vi "PV Telegram return.vi"(4 "String received":string, 5 "Data Typ String":string) -> (0 "error":bool, 1 "Substring":string, 2 "PV Protocol Data out":string)   [LabVIEW 2018, in "Pfeiffer Vacuum.lvlib"]
uses:
  Pfeiffer Vacuum.lvlib
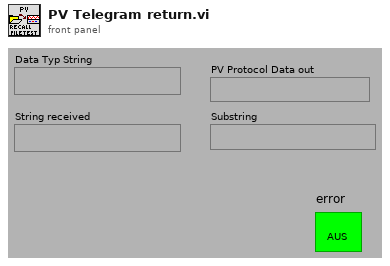
[diagram p1: front panel]
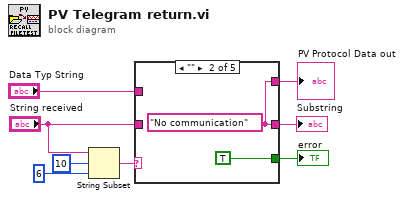
[diagram p0: block diagram]
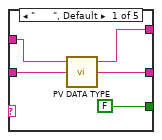
[diagram p2: hidden frame]
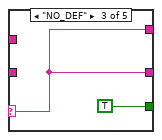
[diagram p3: hidden frame]
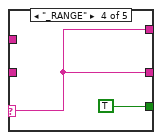
[diagram p4: hidden frame]
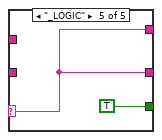
[diagram p5: hidden frame]
diagram:
  n1 = String Subset(string="String received", offset (0)=10 ("Offset (0)"), length (rest)=6 ("Länge")) -> (substring=w6:string)
  n2 = case shown="\"\"" w6 {
    selector: w6 -> [_ _ w16 w18 w20]
    tunnel: [w12 w14 w16 w18 w20] -> w7
    tunnel: "String received" -> [w13 _ _ _ _]
    tunnel: [FALSE TRUE TRUE TRUE TRUE] -> w3
    tunnel: "Data Typ String" -> [w10 _ _ _ _]
    tunnel: [w9 w14 w16 w18 w20] -> w1
    frame "      ", Default {
      n3 = call "PV DATA TYPE.vi"("String in"=w13, "Data Typ String in"=w10) -> ("Substring"=w12:string, "PV Protocol Data out"=w9:string)  [unwired: 2 in]
    }
    frame "" {
      w14 = "No communication"
    }
    frame "NO_DEF" {
    }
    frame "_RANGE" {
    }
    frame "_LOGIC" {
    }
  }
  "Substring" <- w7
  "error" <- w3
  "PV Protocol Data out" <- w1
